vi "34401A DMM Simple Measurement.vi"(0 "VISA resource name":refnum<visa-resource-name>, 1 "Manual Resolution (5.5 Digits)":dbl(ring)=5.5 items=["4.5"=4.5, "5.5"=5.5, "6.5"=6.5], 2 "Manual Range (1.00)":dbl=1.0 format="%_3f", 3 "Enable Auto Range (T: Enable)":bool=TRUE, 5 "Function":u16(ring)=4 items=["DC Voltage", "AC Voltage", "2 - Wire Resistance", "4 - Wire Resistance", "DC Current", "AC Current", "Frequency", "Period", "Continuity", "Diode Checking", "VDC:VDC Ratio", "Temperature", "Capacitance"], 7 "Front/Rear Switch":T1(ring), 11 "error in (no error)":errorcluster) -> (4 "VISA resource name out":refnum<visa-resource-name>, 6 "Measurement":dbl, 15 "error out":errorcluster)   [LabVIEW 2015]
doc: "Use this VI to:\n1- Configure Mode of Measurement & Range/Res.\n2- Take a single measurement\n3- Check for any errors"
uses:
  <instrlib>/Agilent 34401/Public/Data/Read (Single Point).vi
  <instrlib>/Agilent 34401/Agilent 34401.lvlib
panel:
  out "Error Message":string
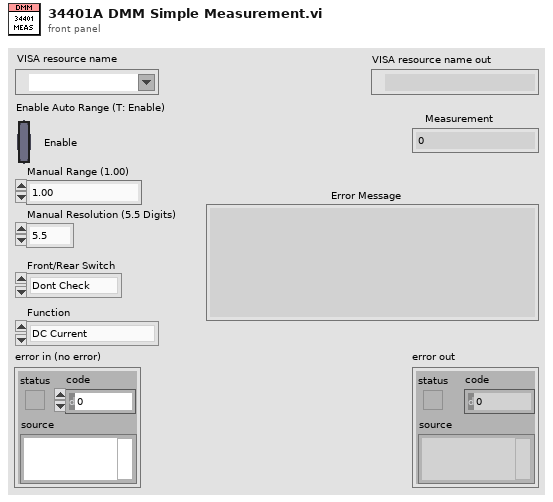
[diagram p1: front panel]
types:
  T1 = enum16{"Dont Check", "Must be Front", "Must be Rear"}
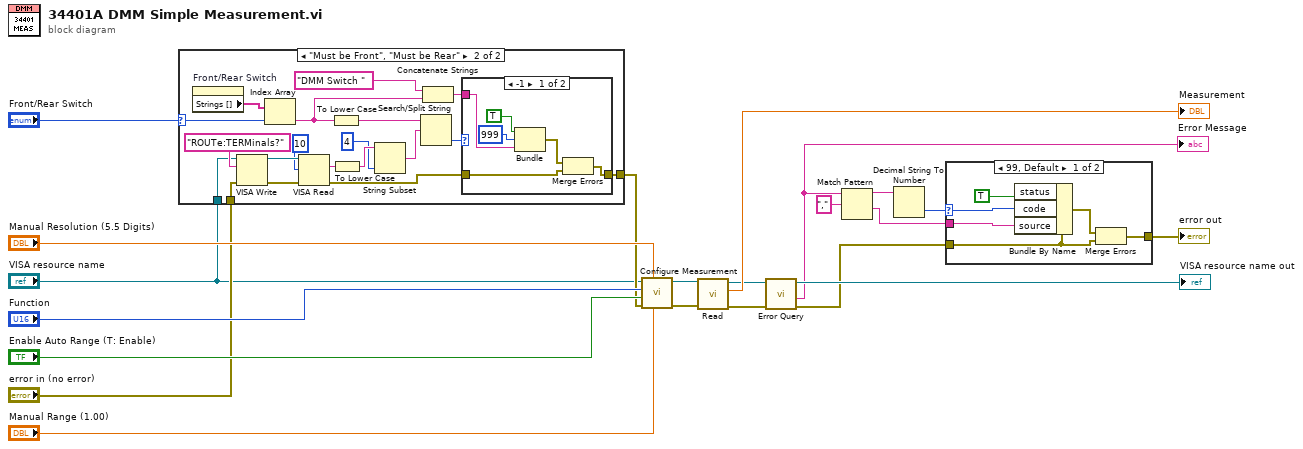
[diagram p0: block diagram]
diagram:
  n1 = case shown="\"Must be Front\", \"Must be Rear\"" "Front/Rear Switch" {
    selector: "Front/Rear Switch" -> [_ w36]
    tunnel: "error in (no error)" -> [w22 w33]
    tunnel: [w22 w28] -> w3
    tunnel: "VISA resource name" -> [_ w27]
    frame "Dont Check", Default {
    }
    frame "Must be Front", "Must be Rear" {
      n2 = property on="Front/Rear Switch" class="Enum (strict)"() -> ("Strings []"=w37:string[])  [unwired: 2 in, 2 out]
      n3 = VISA Write(VISA resource name=w27, write buffer="ROUTe:TERMinals?" ("Query"), error in (no error)=w33) -> (VISA resource name out=w39:refnum<visa-resource-name>, error out=w40:errorcluster)  [unwired: 1 out]
      n4 = Index Array(array=w37, index=w36) -> (element=w30:string)
      n5 = VISA Read(VISA resource name=w39, byte count=u32 10 ("Bytes to Read"), error in (no error)=w40) -> (read buffer=w35:string, error out=w32:errorcluster)  [unwired: 2 out]
      n6 = To Lower Case(string=w30) -> (all lower case string=w26:string)
      n7 = To Lower Case(string=w35) -> (all lower case string=w25:string)
      n8 = String Subset(string=w25, length (rest)=4 ("length (rest)")) -> (substring=w23:string)  [unwired: 1 in]
      n9 = Search/Split String(string=w26, search string/char (-)=w23) -> (offset of match=w34:i32)  [unwired: 1 in, 2 out]
      n10 = Concatenate Strings("DMM Switch ", w30) -> (w29:string)
      n11 = case shown="-1" w34 {
        tunnel: w32 -> [w46 w48]
        tunnel: [w47 w48] -> w28
        tunnel: w29 -> [w44 _]
        frame -1 {
          n12 = Bundle("status"=TRUE, 999, w44) -> (w42:cluster{"status":bool, i32, string})  [unwired: 1 in]
          n13 = Merge Errors(w42, w46) -> (w47:errorcluster)
        }
        frame 0, Default {
        }
      }
    }
  }
  n14 = call <instrlib>:"Configure Measurement.vi"("Manual Range (1.00)"="Manual Range (1.00)", "Manual Resolution (5.5 Digits)"="Manual Resolution (5.5 Digits)", "error in (no error)"=w3, "Enable Auto Range (T: Enable)"="Enable Auto Range (T: Enable)", "Function (0: DC Voltage)"="Function", "VISA resource name"="VISA resource name") -> ("error out"=w20:errorcluster, "VISA resource name out"=w21:refnum<visa-resource-name>)  [unwired: 4 in]
  n15 = call-poly <instrlib>:"Read.vi"("error in (no error)"=w20, "VISA resource name"=w21) -> ("error out"=w18:errorcluster, "Measurement"=→"Measurement":dbl, "VISA resource name out"=w17:refnum<visa-resource-name>)  [unwired: 7 in]
  n16 = call <instrlib>:"Error Query.vi"("error in (no error)"=w18, "VISA resource name"=w17) -> ("error out"=w10:errorcluster, "Error Message"=w15:string, "VISA resource name out"=→"VISA resource name out":refnum<visa-resource-name>)  [unwired: 6 in, 1 out]
  "Error Message" <- w15
  n17 = Match Pattern(string=w15, regular expression=",") -> (before substring=w13:string, after substring=w11:string)  [unwired: 1 in, 2 out]
  n18 = Decimal String To Number(string=w13) -> (number=w12:i32)  [unwired: 2 in, 1 out]
  n19 = case shown="99, Default" w12 {
    selector: w12 -> [w53 _]
    tunnel: w11 -> [w52 _]
    tunnel: w10 -> [w51 w55]
    tunnel: [w49 w55] -> w9
    frame 99, Default {
      n20 = Bundle By Name(cluster=w51, "status"=TRUE, "code"=w53, "source"=w52) -> (w50:errorcluster)
      n21 = Merge Errors(w50, w51) -> (w49:errorcluster)
    }
    frame 0 {
    }
  }
  "error out" <- w9
